vi "Main Tclk.vi"() -> ()   [LabVIEW 2018]
uses:
  <vilib>/Utility/miscctls.llb/LVPoint32TypeDef.ctl
  <vilib>/Utility/miscctls.llb/LVRectTypeDef.ctl
  <vilib>/event_ctls.llb/eventvkey.ctl
  <vilib>/Utility/error.llb/DialogType.ctl
  <vilib>/Analysis/baseanly.llb/Mean (DBL).vi
  <vilib>/DAQmx/read.llb/DAQmx Read (Analog 2D DBL NChan NSamp).vi
  <vilib>/DAQmx/write.llb/DAQmx Write (Digital Bool 1Line 1Point).vi
  <vilib>/DAQmx/create/channels.llb/DAQmx Create Channel (AO-Voltage-Basic).vi
  <vilib>/Utility/file.llb/Read Delimited Spreadsheet (string).vi
  <vilib>/Utility/xml.llb/Read From XML File(string).vi
  <vilib>/measure/madcrms.llb/Basic Averaged DC-RMS for 1 Chan.vi
  Transpose 3D(dbl).vi
  <vilib>/Utility/xml.llb/Write to XML File(string).vi
  <vilib>/DAQmx/create/channels.llb/DAQmx Create Channel (AI-Voltage-Basic).vi
  <vilib>/DAQmx/configure/timing.llb/DAQmx Timing (Sample Clock).vi
  <vilib>/DAQmx/miscellaneous.llb/DAQmx Fill In Error Info.vi
  <vilib>/DAQmx/create/channels.llb/DAQmx Create Channel (DO-Digital Output).vi
  <vilib>/regexp/Match Regular Expression.xnode
  <resource>/objmgr/daqmx.rc
  <vilib>/ptbypt/NI_PtbyPt.lvlib
  <vilib>/Analysis/NI_AALPro.lvlib
  <vilib>/measure/NI_MAPro.lvlib
  <vilib>/Analysis/NI_AALBase.lvlib
  <vilib>/Utility/file.llb/Read From Spreadsheet File (string).vi
panel:
  out "Original WatchDog Mode":u16(ring)=2 items=["Do Nothing", "Send Idle Only", "Watch FIB & SEM", "Watch FIB Only", "Watch SEM Only"]
  in  "FI toggle":bool=TRUE
  out "FRC array":sgl[](array[numeric])
  out "Remaining Y shift frames":u32=1
  out "Remaining X shift frames":u32=1
  out "Last good milling Z voltage (V)":sgl format="%.4f"
  out "FIB CL control band factor":sgl=1.38 format="%.2f"
  out "API timeout":bool
  out "BD1 out of bound":bool
  out "Milling I out of bound":bool
  out "BD2 out of bound":bool
  out "Specimen I out of bound":bool
  in  "WatchDog Mode":u16(ring)=2 items=["Do Nothing", "Send Idle Only", "Watch FIB & SEM", "Watch FIB Only", "Watch SEM Only"]
  out "Detector number":i16
  in  "Reset Watchdog":bool
  in  "Image fit to":u8(ring) items=["Width", "Height"]
  out "Continued fine milling frames":i32
  out "FIB CL control band":sgl=1.38 format="%.2f"
  out "Actual Reheat Parameters":T1
  in  "Start Reheat":bool
  out "FIB suppressor below limit counts":u8
  out "Delta Y array for stop limit":sgl[](array[numeric])
  out "Delta X array for stop limit":sgl[](array[numeric])
  out "FI array for stop limit":sgl[](array[numeric])
  out "Delta Y stop limit array":sgl[](array[numeric])
  out "Delta X stop limit array":sgl[](array[numeric])
  out "FI high stop limit array":sgl[](array[numeric])
  out "FI low stop limit array":sgl[](array[numeric])
  out "FI high warning limit array":sgl[](array[numeric])
  out "FI low warning limit array":sgl[](array[numeric])
  out "Unfreeze":bool
  out "Faraday Cup array":sgl[](array[numeric])
  out "Temp array":sgl[](array[numeric])
  out "FIB single scan":bool
  out "Z removal stop threshold Z(nm)":u8
  out "Mouse down":bool
  out "SEM shutter failed active":bool
  out "SEM shutter warning armed":bool=TRUE
  out "Milling I low limit array":sgl[](array[numeric])
  out "Milling I high limit array":sgl[](array[numeric])
  out "BD2 low limit array":sgl[](array[numeric])
  out "BD2 high limit array":sgl[](array[numeric])
  out "BD1 low limit array":sgl[](array[numeric])
  out "BD1 high limit array":sgl[](array[numeric])
  out "Cycle time array":u32[](array[numeric])
  out "Milling time (s)":sgl
  out "Cycle time est offset array":i16[](array[numeric])
  out "Current DataLog Files":path=path "D:/3D FIB-SEM Files/Current DataLog"
  out "Low Mag SEM on":bool
  out "LM SEM scan time":dbl=0.39999999999999997
  out "SEM HV DataLog Files":path=path "D:/3D FIB-SEM Files/SEM HV DataLog"
  out "PID recovered":bool
  out "Run once":bool
  out "Milling Z realtime (V)":sgl caption="Milling Z (V)" format="%.4g"
  out "Prior Alert Settings":T2={"3D imaging paused alarm"=TRUE, "FIB emission limit warning"=TRUE, "Low limit"=1.4, "High limit"=2.0, "Specimen @ SEM alarm"=TRUE, "Specimen @ FIB alarm "=TRUE, "Beam Dump 1 alarm"=TRUE, "Milling Z voltage alarm"=TRUE, "EHT off alarm"=TRUE, "Detector over scale warning"=TRUE, "Image clipping alarm"=TRUE, "Warning limit (um)"=1.5, "Stop limit (um)"=0.5, "Temperature alarm"=TRUE, "Pause 3D-ING"=FALSE, "Low limit (F)"=65.0, "High limit (F)"=80.0, "Temp limit auto"=TRUE, "Delta (F)"=0.2, "Gradient limit (F/min)"=0.03, "SW error warning"=TRUE, "Focus index warning"=TRUE, "Focus index low limit"=0.1, "Focus index stop limit"=0.0, "Run Auto Stig"=FALSE, "FI low limit auto"=TRUE, "FI stop limit auto"=TRUE} {"Stop limit (um)" format="%.2f"; "Warning limit (um)" format="%.2f"; "Focus index stop limit" format="%_3g"; "Focus index low limit" format="%_3g"; "High limit (F)" format="%.2g"; "Low limit (F)" format="%.2g"}
  out "Faraday Cup high limit array":sgl[](array[numeric])
  out "Faraday Cup low limit array":sgl[](array[numeric])
  out "Specimen I low limit array":sgl[](array[numeric])
  out "Specimen I high limit array":sgl[](array[numeric])
  out "FI low limit array":sgl[](array[numeric])
  out "SEM Specimen I high limit array":sgl[](array[numeric])
  out "SEM Specimen I low limit array":sgl[](array[numeric])
  out "Temp high limit array":sgl[](array[numeric])
  out "Temp low limit array":sgl[](array[numeric])
  out "SEM Specimen I":dbl format="%0.2f"
  out "Milling Z voltage spike":bool
  out "SEM Spec. I spike":bool
  out "Faraday Cup < Milling current":bool
  out "WD Stig Aln tile offsets":T3
  out "Milling I array":sgl[](array[numeric])
  in  "Beam dump display":u8(ring) items=["B.D.1", "B.D.2", "Mill"]
  out "Beam Dump 2 array":sgl[](array[numeric])
  out "FIB CL I out of bound counts":u8
  out "FIB CL I alarm active":bool
  out "AAY Graph scales tiled":cluster{sgl, sgl, sgl, sgl}[][](array[cluster])
  out "AAY Graph tiled":T4(array[cluster])
  out "AAX Graph scales tiled":cluster{sgl, sgl, sgl, sgl}[][](array[cluster])
  out "AAX Graph tiled":T4(array[cluster])
  out "ASY Graph scales tiled":cluster{sgl, sgl, sgl, sgl}[][](array[cluster])
  out "ASY Graph tiled":T4(array[cluster])
  out "ASX Graph tiled":T4(array[cluster])
  out "ASX Graph scales tiled":cluster{sgl, sgl, sgl, sgl}[][](array[cluster])
  out "AF Graph scales tiled":cluster{sgl, sgl, sgl, sgl}[][](array[cluster])
  out "Auto Focus Graph tiled":T4(array[cluster])
  out "Skip Steps tiled":u8[][](array[numeric])
  out "Focus Index array tiled":sgl[][][][](array[numeric])
  out "FI array tiled":sgl[][][](array[numeric])
  out "FI grid array tiled":sgl[][][][][](array[numeric])
  out "Focus Index tiled":sgl[][](array[numeric])
  out "AlnX array tiled":sgl[][][](array[numeric])
  out "AlnY array tiled":sgl[][][](array[numeric])
  out "StigY array tiled":sgl[][][](array[numeric])
  out "StigX array tiled":sgl[][][](array[numeric])
  out "SEM Mid Mag Scan Parameters":T5={"X size (um)"=200.0, "Y size (um)"=200.0, "X center (um)"=0.0, "Y center (um)"=0.0, "X size (V)"=8.081220354352679, "X size auto"=TRUE, "X stig"=[[0.0]], "Y stig"=[[0.0]], "X aln"=[[0.0]], "Y aln"=[[0.0]], "Scan rate (Hz)"=1000000, "Oversampling"=50, "Oversampling auto"=TRUE, "Frame line rampdown ratio"=0.1, "Pixel size (nm)"=10.0, "WD (mm)"=[[3.0]], "X tiles"=1, "Y tiles"=1, "Overlap (um)"=1.0, "Interlaced"=TRUE, "dX (um)"=[0.0], "dY (um)"=[0.0], "Frames"=1} {"dY (um)" format="%.1f"; "dX (um)" format="%.1f"; "Frames" min=1 step=1; "WD (mm)" format="%.1f"; "Y aln" format="%.1f"; "X aln" format="%.1f"; "Y stig" format="%.1f"; "X stig" format="%.1f"; "Overlap (um)" min=0; "Y tiles" min=1; "X tiles" min=1; "X size (um)" format="%.2f"; "Y size (um)" format="%.2f"; "Frame line rampdown ratio" min=0 max=1 step=0.05 format="%.2g"; "X center (um)" step=1.0 format="%.2f"; "Y center (um)" step=1.0 format="%.2f"; "X size (V)" format="%_4g"; "Scan rate (Hz)" max=4000000 step=100000 format="%.2e"}
  out "SEM Low Mag Scan Parameters":T5={"X size (um)"=20.0, "Y size (um)"=20.0, "X center (um)"=0.0, "Y center (um)"=0.0, "X size (V)"=6.190428211586902, "X size auto"=TRUE, "X stig"=[[0.0]], "Y stig"=[[0.0]], "X aln"=[[0.0]], "Y aln"=[[0.0]], "Scan rate (Hz)"=10000000, "Oversampling"=5, "Oversampling auto"=TRUE, "Frame line rampdown ratio"=0.1, "Pixel size (nm)"=10.0, "WD (mm)"=[[3.0]], "X tiles"=1, "Y tiles"=1, "Overlap (um)"=1.0, "Interlaced"=TRUE, "dX (um)"=[0.0], "dY (um)"=[0.0], "Frames"=1} {"dY (um)" format="%.1f"; "dX (um)" format="%.1f"; "Frames" min=1 step=1; "WD (mm)" format="%.1f"; "Y aln" format="%.1f"; "X aln" format="%.1f"; "Y stig" format="%.1f"; "X stig" format="%.1f"; "Overlap (um)" min=0; "Y tiles" min=1; "X tiles" min=1; "X size (um)" format="%.2f"; "Y size (um)" format="%.2f"; "Frame line rampdown ratio" min=0 max=1 step=0.05 format="%.2g"; "X center (um)" step=1.0 format="%.2f"; "Y center (um)" step=1.0 format="%.2f"; "X size (V)" format="%_4g"; "Scan rate (Hz)" max=4000000 step=100000 format="%.2e"}
  in  "Tiled scan inputs":T6={"HW Config"={"SEM X coil"="SEM-X", "SEM Y coil"="SEM-Y", "Detectors"="Detectors", "Det min (V)"=-10.0, "Det max (V)"=10.0, "Eanable COM"=TRUE, "COM port"="COM1", "Detector FIB-NI auto switch"="FIB/port0/line0", "Machine Type"=0, "Machine ID"="Feiss/Sigma-01-42", "SEM Max FOV (um)"=350.0}, "Det Info"={"Brightness A"=40.0, "Contrast A"=26.0, "Detector B name"="ESB @ 1.0 kV", "Brightness B"=40.0, "Contrast B"=40.0, "Detector C name"="PMT @ 6.0", "Detector D name"="Detector D"}, "SEM Scan Parameters"={"X size (um)"=20.0, "Y size (um)"=20.0, "X center (um)"=0.0, "Y center (um)"=0.0, "X size (V)"=6.190428211586902, "X size auto"=TRUE, "X stig"=[[0.0]], "Y stig"=[[0.0]], "X aln"=[[0.0]], "Y aln"=[[0.0]], "Scan rate (Hz)"=10000000, "Oversampling"=5, "Oversampling auto"=TRUE, "Frame line rampdown ratio"=0.1, "Pixel size (nm)"=10.0, "WD (mm)"=[[3.0]], "X tiles"=1, "Y tiles"=1, "Overlap (um)"=1.0, "Interlaced"=TRUE, "dX (um)"=[0.0], "dY (um)"=[0.0], "Frames"=1}, "SEM Options"={"GetInfo"=TRUE, "Set Det A para"=TRUE, "Set WD"=FALSE, "Set Mag"=TRUE, "Set stig"=FALSE, "Set aln"=FALSE, "Display"=TRUE, "Save"=TRUE, "8-bit"=TRUE, "Detector A"=TRUE, "Detector B"=FALSE, "Detector C"=FALSE, "Detector D"=FALSE, "Inverse A"=FALSE, "Inverse B"=FALSE, "Inverse C"=FALSE, "Inverse D"=FALSE, "Inverse PNG"=TRUE, "Freeze"=TRUE, "PNG only"=FALSE, "Upload"=FALSE, "Delete after upload"=FALSE}, "Focus Index Options"={"Keep aspect ratio"=FALSE, "Show Focus Index"=TRUE, "Focus Index primary grid center"=TRUE, "X Grids"=[[0]], "Y Grids"=[[0]], "Primary X index"=[[0]], "Primary Y index"=[[0]]}, "File Information"={"File path"=path "E:/Images", "Notes"="", "Save recipe"=FALSE, "Load recipe"=FALSE, "Sample ID"=""}, "Milling para"={"X resolution"=4096, "Y resolution"=125001, "X offset (um)"=0.0, "Y offset (um)"=0.0, "X center (um)"=0.0, "Y center (um)"=0.0, "X size (um)"=250.0, "Y size (um)"=250.0, "UL-Ang"=90.0, "UR-Ang"=90.0, "Line milling time (s)"=5.0, "Z-step (nm)"=2.0, "Lines auto pause"=1, "Auto pause"=FALSE, "Mill from Bottom"=FALSE, "FIB FOV (um)"=500.0, "Auto Profile"=FALSE, "Mill start from Last"=FALSE, "FIB PID on"=FALSE, "FIB PID reset"=TRUE, "FIB PID measured"=0, "FIB PID target"=0.0, "FIB PID target slope"=0.0, "FIB PID P"=0.001, "FIB PID I"=0.01, "FIB PID D"=0.0, "Emission (uA)"=1.36, "Suppressor (V)"=50.0, "Auto reheat"=FALSE}, "Additional Info"={"Restart flag"=0, "Stage move flag"=0}} {"Milling para"."Suppressor (V)" step=0.1 format="%.1g"; "Milling para"."Emission (uA)" step=0.1 format="%.2g"; "Milling para"."FIB PID measured" items=["Spec.", "B.D. 1", "B.D. 2", "Mill", "Spec. +"]; "Milling para"."FIB PID target slope" min=-1 max=1 step=0.1; "Milling para"."UR-Ang" format="%.2f"; "Milling para"."UL-Ang" format="%.2f"; "Milling para"."Y offset (um)" step=0.02 format="%.3g"; "Milling para"."X offset (um)" step=1 format="%.3g"; "Milling para"."FIB FOV (um)" format="%.3g"; "Milling para"."Line milling time (s)" format="%.1f"; "Milling para"."Y center (um)" format="%#.3g"; "Milling para"."X center (um)" format="%#.3g"; "SEM Scan Parameters"."dY (um)" format="%.1f"; "SEM Scan Parameters"."dX (um)" format="%.1f"; "SEM Scan Parameters"."Frames" min=1 step=1; "SEM Scan Parameters"."WD (mm)" format="%.1f"; "SEM Scan Parameters"."Y aln" format="%.1f"; "SEM Scan Parameters"."X aln" format="%.1f"; "SEM Scan Parameters"."Y stig" format="%.1f"; "SEM Scan Parameters"."X stig" format="%.1f"; "SEM Scan Parameters"."Overlap (um)" min=0; "SEM Scan Parameters"."Y tiles" min=1; "SEM Scan Parameters"."X tiles" min=1; "SEM Scan Parameters"."X size (um)" format="%.2f"; "SEM Scan Parameters"."Y size (um)" format="%.2f"; "SEM Scan Parameters"."Frame line rampdown ratio" min=0 max=1 step=0.05 format="%.2g"; "SEM Scan Parameters"."X center (um)" step=1.0 format="%.2f"; "SEM Scan Parameters"."Y center (um)" step=1.0 format="%.2f"; "SEM Scan Parameters"."X size (V)" format="%_4g"; "SEM Scan Parameters"."Scan rate (Hz)" max=4000000 step=100000 format="%.2e"; "HW Config"."Machine Type" items=["Feiss", "NVision"]}
  out "Focus index stop trigger active":bool
  out "FI below limit counts":u8
  out "FIB emission below limit counts":u8
  out "Turn FIB Gun on":bool
  out "Reheat log file":path
  out "FIB HV DataLog Files":path=path "D:/3D FIB-SEM Files/FIB HV DataLog"
  out "Email recipents file":path=path "D:/3D FIB-SEM Files/Email alert recipients.txt"
  out "dat to csv and xml":bool
  in  "Aln Options":enum16{"Defaut", "Aln X", "Aln Y"}(ring)
  in  "Delta Z mode":u8
  out "Delta Z array":sgl[](array[numeric])
  out "Milling Z voltage array":sgl[](array[numeric])
  in  "Specimen current toggle":bool=TRUE
  out "SEM Specimen I array":sgl[](array[numeric])
  in  "SW date":string="01/02/2022"
  out "Smart upload fail":bool
  out "Re-engage warning armed":bool=TRUE
  out "Y shift from last":dbl
  out "X shift from last":dbl
  out "Reheat from last":bool
  out "Last re-engage count":u8
  out "Re-engage Delta X array":dbl[](array[numeric])
  out "Beam dump at zero":bool
  in  "Pause for reheat":bool
  out "MM SEM scan time":dbl=400.0
  out "Focus index warning active":bool
  out "Temperature warning active":bool
  out "FIB emission limit warning active":bool
  out "3D image paused active":bool
  out "SW error warning active":bool
  in  "Delta Y toggle":bool
  in  "Delta X toggle":bool
  out "Delta Y sum array":sgl[](array[numeric])
  out "Delta X sum array":sgl[](array[numeric])
  out "Focus index array":sgl[](array[numeric])
  out "Delta image array":sgl[](array[numeric])
  out "Delta Y array":sgl[](array[numeric])
  out "Delta X array":sgl[](array[numeric])
  out "3D FIB-SEM Files":path=path "D:/3D FIB-SEM Files"
  in  "Load recipe":bool
  in  "Read recipe path":path
  out "SEM scan time":dbl=10.999999999999998
  out "Trapezoidal":cluster{"X":i16, "Y":i16}[](array[cluster])=[{"X"=128, "Y"=128}, {"X"=384, "Y"=128}, {"X"=384, "Y"=384}, {"X"=128, "Y"=384}, {"X"=128, "Y"=128}]
  out "Last Det B Low Mag":path=path "D:/3D FIB-SEM Files/Last DetB LM image.png"
  out "Last Det A Low Mag":path=path "D:/3D FIB-SEM Files/Last DetA LM image.png"
  out "Last FIB zoom pre image":path=path "D:/3D FIB-SEM Files/Last FIB zoom pre image.png"
  out "Last FIB image":path=path "D:/3D FIB-SEM Files/Last FIB image.png"
  in  "Recipe input":T7={"SEM Scan Parameters"={"X size (um)"=80.0, "Y size (um)"=80.0, "X center (um)"=0.0, "Y center (um)"=0.0, "X size (V)"=3.2324881417410714, "X size auto"=TRUE, "X stig"=[[0.0]], "Y stig"=[[0.0]], "X aln"=[[0.0]], "Y aln"=[[0.0]], "Scan rate (Hz)"=10000000, "Oversampling"=2, "Oversampling auto"=TRUE, "Frame line rampdown ratio"=0.1, "Pixel size (nm)"=8.0, "WD (mm)"=[[3.0]], "X tiles"=1, "Y tiles"=1, "Overlap (um)"=2.0, "Interlaced"=TRUE, "dX (um)"=[0.0], "dY (um)"=[0.0], "Frames"=1}, "Detector Information"={"Brightness A"=35.0, "Contrast A"=28.0, "Detector B name"="ESB @ 600 V", "Brightness B"=30.0, "Contrast B"=38.0, "Detector C name"="Detector C", "Detector D name"="Detector D"}, "SEM Options"={"GetInfo"=TRUE, "Set Det A para"=TRUE, "Set WD"=FALSE, "Set Mag"=TRUE, "Set stig"=FALSE, "Set aln"=FALSE, "Display"=TRUE, "Save"=TRUE, "8-bit"=TRUE, "Detector A"=TRUE, "Detector B"=TRUE, "Detector C"=FALSE, "Detector D"=FALSE, "Inverse A"=FALSE, "Inverse B"=FALSE, "Inverse C"=FALSE, "Inverse D"=FALSE, "Inverse PNG"=TRUE, "Freeze"=TRUE, "PNG only"=FALSE, "Upload"=FALSE, "Delete after upload"=FALSE}, "Focus Index Options"={"Keep aspect ratio"=FALSE, "Show Focus Index"=TRUE, "Focus Index primary grid center"=TRUE, "X Grids"=[[1]], "Y Grids"=[[1]], "Primary X index"=[[1]], "Primary Y index"=[[1]]}, "Image fit to"=0, "File Information"={"File path"=path "E:/Images", "Notes"="", "Save recipe"=FALSE, "Load recipe"=FALSE, "Sample ID"=""}, "Low mag SEM"={"Low mag scan"=TRUE, "Prior to main scan"=FALSE, "Low mag interval"=1, "Low mag scan FOV (micron)"=300.0, "Low mag scan rate (Hz)"=1000000, "Show HM box"=TRUE}, "Mid Mag SEM"={"Mid mag scan"=FALSE, "Prior to main scan"=FALSE, "Mid mag interval"=500, "X size (um)"=200.0, "Y size (um)"=200.0, "X center (um)"=0.0, "Y center (um)"=0.0, "Mid mag scan rate (Hz)"=1000000, "Pixel size (nm)"=10.0, "Show MM box"=TRUE}, "FIB-SEM Angle"=90.0, "Milling para"={"X resolution"=4096, "Z resolution"=125001, "X offset (um)"=0.0, "Z offset (um)"=0.0, "X center (um)"=0.0, "Z center (um)"=0.0, "X size (um)"=250.0, "Z size (um)"=250.0, "UL-Ang"=90.0, "UR-Ang"=90.0, "Line milling time (s)"=5.0, "Z-step (nm)"=2.0, "Lines auto pause"=1, "Auto pause"=FALSE, "Mill from Bottom"=FALSE, "FIB FOV (um)"=500.0, "Auto Profile"=FALSE, "Mill start from Last"=FALSE, "FIB PID on"=FALSE, "FIB PID reset"=FALSE, "FIB PID measured"=0, "FIB PID target"=0.0, "FIB PID target slope"=0.0, "FIB PID P"=0.001, "FIB PID I"=0.01, "FIB PID D"=0.0, "Emission (uA)"=1.36, "Suppressor (V)"=50.0, "Auto reheat"=FALSE}, "FI Detector"=0, "Auto Optimzation"=TRUE, "Images per Auto Optimization"=200, "AF Range (nm)"=1800.0, "AF Steps"=7, "AS Range (%)"=0.4000000059604645, "AS Steps"=7, "AA Range (%)"=6.0, "AA Steps"=7, "X shift (nm/frame)"=0.0, "Y shift (nm/frame)"=0.0, "FIB Y zoom pixel (nm)"=20.0, "Mail server"="mail.hhmi.org", "Email Alert Recipents"=["xuc@janelia.hhmi.org"], "Alert Settings"={"3D imaging paused alarm"=TRUE, "FIB emission limit warning"=TRUE, "Low limit"=1.38, "High limit"=2.0, "Specimen @ SEM alarm"=TRUE, "FIB CL current alarm"=TRUE, "Beam Dump 1 alarm"=TRUE, "Milling Z voltage alarm"=TRUE, "EHT off alarm"=TRUE, "Detector over scale warning"=TRUE, "Image clipping alarm"=FALSE, "Warning limit (um)"=1.5, "Stop limit (um)"=0.5, "Temperature alarm"=TRUE, "Pause 3D-ING"=FALSE, "Low limit (F)"=65.0, "High limit (F)"=80.0, "Temp limit auto"=TRUE, "Delta (F)"=0.2, "Gradient limit (F/min)"=0.03, "SW error warning"=TRUE, "Focus index warning"=TRUE, "Focus index low limit"=0.1, "Focus index stop limit"=0.0, "Run Auto Stig"=FALSE, "FI low limit auto"=TRUE, "FI stop limit auto"=TRUE}, "Reheat Parameters"={"Filament I (A)"=3.0, "Reheat time (s)"=45.0, "Emission (uA)"=1.5, "Calculate V/I slope"=TRUE, "Pre-calc delay (min)"=5.0, "Disable Reheat Retries"=FALSE, "Restore Voltages"=TRUE}, "Start FIB HV DataLog"=TRUE, "Interval (s)"=60} {"Milling para"."Suppressor (V)" step=0.1 format="%.1g"; "Milling para"."Emission (uA)" step=0.1 format="%.2g"; "Milling para"."FIB PID measured" items=["Spec.", "B.D. 1", "B.D. 2", "Mill", "Spec. +"]; "Milling para"."FIB PID target slope" min=-1 max=1 step=0.1; "Milling para"."UR-Ang" format="%.2f"; "Milling para"."UL-Ang" format="%.2f"; "Milling para"."Z offset (um)" step=0.02 format="%.3g"; "Milling para"."X offset (um)" step=1 format="%.3g"; "Milling para"."FIB FOV (um)" format="%.3g"; "Milling para"."Line milling time (s)" format="%.1f"; "Milling para"."Z center (um)" format="%#.3g"; "Milling para"."X center (um)" format="%#.3g"; "Alert Settings"."Stop limit (um)" format="%.2f"; "Alert Settings"."Warning limit (um)" format="%.2f"; "Alert Settings"."Focus index stop limit" format="%_3g"; "Alert Settings"."Focus index low limit" format="%_3g"; "Alert Settings"."High limit (F)" format="%.2g"; "Alert Settings"."Low limit (F)" format="%.2g"; "Alert Settings"."High limit" format="%.2f"; "Alert Settings"."Low limit" format="%.2f"; "SEM Scan Parameters"."dY (um)" format="%.1f"; "SEM Scan Parameters"."dX (um)" format="%.1f"; "SEM Scan Parameters"."Frames" min=1 step=1; "SEM Scan Parameters"."WD (mm)" format="%.1f"; "SEM Scan Parameters"."Y aln" format="%.1f"; "SEM Scan Parameters"."X aln" format="%.1f"; "SEM Scan Parameters"."Y stig" format="%.1f"; "SEM Scan Parameters"."X stig" format="%.1f"; "SEM Scan Parameters"."Overlap (um)" min=0; "SEM Scan Parameters"."Y tiles" min=1; "SEM Scan Parameters"."X tiles" min=1; "SEM Scan Parameters"."X size (um)" format="%.2f"; "SEM Scan Parameters"."Y size (um)" format="%.2f"; "SEM Scan Parameters"."Frame line rampdown ratio" min=0 max=1 step=0.05 format="%.2g"; "SEM Scan Parameters"."X center (um)" step=1.0 format="%.2f"; "SEM Scan Parameters"."Y center (um)" step=1.0 format="%.2f"; "SEM Scan Parameters"."X size (V)" format="%_4g"; "SEM Scan Parameters"."Scan rate (Hz)" max=4000000 step=100000 format="%.2e"; "Reheat Parameters"."Pre-calc delay (min)" format="%.2f"; "Reheat Parameters"."Emission (uA)" format="%.1f"; "Reheat Parameters"."Filament I (A)" format="%.2f"; "Reheat Parameters"."Reheat time (s)" format="%.1f"; "Image fit to" items=["Width", "Height"]; "Mid Mag SEM"."X center (um)" step=1.0 format="%.4f"; "Mid Mag SEM"."Y center (um)" step=1.0 format="%.4f"; "Mid Mag SEM"."Mid mag interval" min=1 step=1; "Mid Mag SEM"."Mid mag scan rate (Hz)" max=4000000 step=100000 format="%.2e"; "FIB Y zoom pixel (nm)" format="%.1g"; "X shift (nm/frame)" step=0.1; "Y shift (nm/frame)" step=0.1; "FI Detector" items=["A", "B", "C", "D"]; "Low mag SEM"."Low mag interval" min=1 step=1; "Low mag SEM"."Low mag scan rate (Hz)" max=4000000 step=100000 format="%.2e"; "Low mag SEM"."Low mag scan FOV (micron)" step=50.0; "FIB-SEM Angle" min=0.0 max=90.0}
  out "Last milling snapshot":path=path "D:/3D FIB-SEM Files/Last FIB milling snapshot.xml"
  out "Last FIB recipe":path=path "D:/3D FIB-SEM Files/Last FIB recipe.csv"
  in  "FIB time lapse":bool
  out "Beam Dump 1 array":sgl[](array[numeric])
  out "Specimen I array":sgl[](array[numeric])
  in  "Detector Information":T8={"Brightness A"=35.0, "Contrast A"=28.0, "Detector B name"="ESB @ 600 V", "Brightness B"=30.0, "Contrast B"=38.0, "Detector C name"="Detector C", "Detector D name"="Detector D"}
  out "X full scale (V)":sgl=14.142136
  out "error out":errorcluster
  out "HW config items":string[](array[string])=["Machine ID", "Machine type", "SEM maximum FOV (um)", "Detector min (V)", "Detector max (V)", "Brightness A", "Contrast A", "Detector B name", "Brightness B", "Contrast B"]
  out "Y offset pre (um)":dbl
  out "X offset pre (um)":dbl
  out "SEM FOV":dbl=350.0
  in  "Off":bool
  in  "3D FIB-SEM":bool
  in  "SEM HW Config":T9={"SEM X coil"="SEM-X", "SEM Y coil"="SEM-Y", "Detectors A&B"="Detectors", "Det min (V)"=-10.0, "Det max (V)"=10.0, "Eanable COM"=TRUE, "COM port"="COM1", "Detector FIB-NI auto switch"="FIB/port0/line2", "Machine Type"=2, "Machine ID"="Jeiss6/Merlin-xxxx", "SEM Max FOV (um)"=350.0} {"Machine Type" items=["Feiss", "NVision"]}
  out "Low blanked":bool
  out "Milling mode":T10(ring)=enum."FIB"
  out "Machine Type":u8=2
  in  "Reset":bool
  in  "Status Tabs":T11(tab)
  out "FRC resolution":sgl caption="FRC (nm)" format="%.1f"
  out "Beam Dump 2 (nA)":sgl caption="B.D.2" format="%.2g"
  out "Temp range (F)":sgl caption="Range (F)" format="%.2g"
  out "Lines auto pause":u16=1
  out "FIB slice #":u32
  out "Line progress":u8(slide) scale=0.0..100.0
  out "Total\nprogress":u8(slide) scale=0.0..100.0
  out "SEM Status":T12={"AO SampClk.MaxRate"=100000000.0, "AI SampClk.MaxRate"=100000000.0, "AO rate"=10000000.0, "Scan speed"=4, "Detector #"=2, "X min (V)"=-10.0, "X max (V)"=10.0, "X min index"=0, "X max index"=1023, "AO multiline"=512, "Decimating factor"=2, "AvailSampPerChan"=0, "AO scan line"=0, "Total pixels recorded"=0, "Lines scanned"=0, "Scan time (m)"=0.0, "Scan time (s)"=10.999999999999998, "Remaining time (m)"=0, "Remaining time (s)"=0, "SEM Spec. I (nA)"=0.0, "Frame"=1, "X tile"=0, "Y tile"=0} {"Frame" min=1 step=1; "Y tile" min=1; "X tile" min=1; "SEM Spec. I (nA)" format="%.2g"; "AvailSampPerChan" scale=0.0..32000000.0; "Scan time (s)" format="%.2f"; "Total pixels recorded" scale=-1.0..3125000.0; "Scan speed" scale=1.0..15.0; "AO rate" format="%#_3e"}
  out "Rect Milling Post-pause Lines":u16
  out "Temp (F)":sgl=84.375 format="%.2g"
  out "Faraday Cup (nA)":sgl caption="Faraday" format="%.2g"
  out "Specimen I (nA)":sgl caption="Spec." format="%.2g"
  out "Beam Dump 1 (nA)":sgl caption="B.D.1" format="%.2g"
  out "Temp gradient (F/min)":dbl caption="Gradient (F/min)" format="%#_5g"
  out "Focus Index":sgl format="%#_3g"
  out "Delta image":sgl caption="DImage" format="%#_3g"
  out "Delta Y":sgl caption="DY (nm)" format="%.1f"
  out "Delta X":sgl caption="DX (nm)" format="%.1f"
  out "Delta Z (nm)":sgl caption="DZ (nm)" format="%.1f"
  out "Align failed array":bool[][](array[boolean]) caption="Align failed"
  out "Milling I (nA)":sgl caption="Mill" format="%.2g"
  out "Est. cycle time (s)":u32=16 caption="Estimate"
  out "Actual cycle time (s)":u32 caption="Actual"
  out "Median cycle time (s)":u32 caption="Median"
  out "Overhead (s)":sgl=5.0
  out "Daily Z removal (um)":sgl=10.8 format="%.2f"
  out "Median cycle time est offset (s)":i16 caption="Offset"
  out "Timeout threshold (s)":u32=36
  out "LM overhead":u32
  out "MM overhead":u32
  out "SEM Parameters":T13={"Detector A"="InLens", "Detector B"="Detector B", "Brightness A"=0.0, "Contrast A"=0.0, "Brightness B"=0.0, "Contrast B"=0.0, "Magnification"=0.0, "Pixel size"=0.0, "Working distance"=0.0, "EHT"=0.0, "Aperture"=0, "High current mode"=0, "Probe current"=0.0, "Scan rotation"=0.0, "Chamber vac"=0.0, "Gun vac"=0.0, "Beam shift X"=0.0, "Beam shift Y"=0.0, "Stig X"=0.0, "Stig Y"=0.0, "Alignment X"=0.0, "Alignment Y"=0.0, "Stage X"=0.0, "Stage Y"=0.0, "Stage Z"=0.0, "Stage T"=0.0, "Stage R"=0.0, "Stage M"=0.0} {"Gun vac" format="%.2e"; "Chamber vac" format="%.2e"}
  out "Image Focus Index":T14
  in  "Image Focus Index Array":T15
  out "Last good FI":sgl
  out "SEM HV Data Output":T16={"Ext Target (V)"=3000.0, "Ext Actual (V)"=3000.0, "Fil Age (hr)"=268.2492, "Ext I Actual (uA)"=200.0, "Fil I Target (A)"=2.0, "Fil I Actual (A)"=2.0, "Liner Target (V)"=8000.0, "Liner Actual (V)"=8000.0, "EHT Target (V)"=3000.0, "EHT Actual (V)"=3000.0, "Supp Actual (V)"=300.0, "Supp Monitor (V)"=0.0, "Gun Vac (Torr)"=1.6651377e-09, "Sys Vac (Torr)"=3.000248e-06} {"Sys Vac (Torr)" format="%.2e"; "Gun Vac (Torr)" format="%.2e"; "Supp Monitor (V)" format="%.1f"; "Liner Actual (V)" format="%.1f"; "Fil I Actual (A)" format="%.3f"; "Ext Actual (V)" format="%.1f"; "Supp Actual (V)" format="%.1f"; "EHT Actual (V)" format="%.1f"; "EHT Target (V)" format="%.1f"; "Liner Target (V)" format="%.1f"; "Fil I Target (A)" format="%.3f"; "Fil Age (hr)" format="%.2f"; "Ext I Actual (uA)" format="%.1f"; "Ext Target (V)" format="%.1f"}
  out "Capella HV Data Output":T17={"Filament (A)"=0.0, "Accelerator Target (V)"=30000.0, "Accelerator Actual (V)"=30021.123, "Extrator Target (V)"=-6400.0, "Extrator Actual (V)"=-6400.0, "Emission Target (uA)"=1.5, "Emission Actual (uA)"=1.545424, "Suppressor (V)"=848.9451, "Faraday I (nA)"=0.0, "Lens1 Target (V)"=-5110.0, "Lens1 Actual (V)"=-5109.8203, "Lens2 Target (V)"=14275.0, "Lens2 Actual (V)"=14265.08, "Gun Vac (Torr)"=9.053087e-09, "Column Vac (Torr)"=2.0494905e-08, "Tip Lifetime (uAhr)"=537.6667} {"Column Vac (Torr)" format="%.2e"; "Gun Vac (Torr)" format="%.2e"; "Lens2 Actual (V)" format="%.1f"; "Lens1 Actual (V)" format="%.1f"; "Emission Actual (uA)" format="%.3f"; "Extrator Actual (V)" format="%.1f"; "Tip Lifetime (uAhr)" format="%.2f"; "Lens2 Target (V)" format="%.1f"; "Lens1 Target (V)" format="%.1f"; "Faraday I (nA)" format="%.3f"; "Suppressor (V)" format="%.1f"; "Emission Target (uA)" format="%.3f"; "Extrator Target (V)" format="%.1f"; "Accelerator Actual (V)" format="%.1f"; "Accelerator Target (V)" format="%.1f"; "Filament (A)" format="%.2f"}
  out "HV Data Output":T18 {"Tip Lifetime (hr)" format="%.2f"; "Lens2I (uA)" format="%.3f"; "Lens2 (V)" format="%.1f"; "Lens1I (uA)" format="%.3f"; "Lens1 (V)" format="%.1f"; "SuppI (uA)" format="%.3f"; "Suppressor (V)" format="%.1f"; "Emission (uA)" format="%.3f"; "Extrator (V)" format="%.1f"; "AccI (uA)" format="%.3f"; "Accelerator (V)" format="%.1f"; "Filament (A)" format="%.2f"}
  out "FIB HV target matched":bool=TRUE
  in  "FIB mill target by spec. I (nA)":sgl format="%.2g"
  out "FIB profile X center (um)":dbl
  out "PID feedback mean (V)":sgl caption="==> mean (V)" format="%.4f"
  out "PID feedback (V)":sgl format="%.4f"
  out "Re-engage Files":path=path "D:/3D FIB-SEM Files/Re-engage"
  out "Milling Z voltage (V)":sgl format="%.4f"
  out "Faraday Cup before mill":sgl caption="Faraday Cup" format="%.3g"
  out "FIB profile Y center (um)":dbl
  out "FIB Parameters":T19 {"FIB stig Y" format="%.2g"; "FIB stig X" format="%.2g"; "FIB emission (uA)" format="%.2f"}
  out "FIB Status":T20 {"Fetch backlog" format="%#_6p"; "Actual sample rate" format="%#_6p"; "Actual scan rate" format="%#_4p"}
  out "Reheat Output":T21 {"Initial suppressor (V)" format="%.1f"; "Initial emission (uA)" format="%.3f"; "V/I Slope" format="%.2f"}
  out "Faraday cup I low":bool
  out "Re-engage Y shift array":dbl[](array[numeric])
  out "Re-engage time":timestamp
  out "Pre-reheat X center (um)":dbl format="%.4f"
  out "Re-engage X shift (um)":dbl format="%.4f"
  in  "Cancel Auto re-engage":bool
  out "Auto re-engage":bool
  out "Pre-reheat FI":dbl format="%.3g"
  out "Re-engage Y shift (um)":dbl format="%.4f"
  out "Re-engage Y stig shift":dbl format="%.4f"
  out "Pre-reheat Y center (um)":dbl format="%.4f"
  in  "a":dbl=0.78 format="%.2f"
  in  "b":dbl=1.0 format="%.2f"
  out "Recovered counts":u8
  out "Image shift search failed":bool
  out "Pre-reheat time":timestamp
  out "Re-engage counts":u8
  out "Re-engage Delta Y array":dbl[](array[numeric])
  out "Re-engage X shift array":dbl[](array[numeric])
  out "Pre-reheat Y stig":sgl[][](array[numeric]) format="%#_3g"
  out "Re-engage cancelled":bool
  out "Pre-reheat FIB PID target":sgl
  out "Mouse Down Coords":T22={"Horizontal"=839, "Vertical"=480}
  in  "FIB Imaging":bool
  in  "FIB HW Config":T23={"FIB X coil"="FIB/ao0", "FIB Y coil"="FIB/ao1", "Beam blank"="FIB/port0/line0", "FIB Ext Scan"="FIB/port0/line1", "Detector"="FIB/ai1", "Shutter Drive"="Log/ao0"}
  in  "Config Tabs":T24(tab)=enum."SEM"
